vi "UHR-Fleezers Control (host) -TL FB Corrected Ronen.vi"(0 "Tab Control":T5(tab)=enum."DAQ AI") -> ()   [LabVIEW 2013] (continued)
        n1853 = Array Subset(array=w2653, index (col)=0 ("index"), length (col)=w2642) -> (w2652:dbl[][])  [unwired: 2 in]
        n1854 = Array Subset(array=w2653, index (col)=w2642) -> (w2650:dbl[][])  [unwired: 3 in]
        n1855 = Array Subset(array=w2727, index (col)=0 ("index"), length (col)=w2642) -> (w2726:dbl[][])  [unwired: 2 in]
        n1856 = Array Subset(array=w2727, index (col)=w2642) -> (w2724:dbl[][])  [unwired: 3 in]
        n1857 = Array Subset(array=w2710, index (col)=0 ("index"), length (col)=w2642) -> (w2715:dbl[][])  [unwired: 2 in]
        n1858 = Array Subset(array=w2710, index (col)=w2642) -> (w2713:dbl[][])  [unwired: 3 in]
        n1859 = for {
          tunnel: w2722 -> [w2764] mode=indexing
          tunnel: [w2763] -> w2721 mode=indexing
          workers-P: _ -> [_]
          n1860 = Reverse 1D Array(array=w2764) -> (reversed array=w2763:dbl[])
        }
        n1861 = for {
          tunnel: w2708 -> [w2760] mode=indexing
          tunnel: [w2759] -> w2707 mode=indexing
          workers-P: _ -> [_]
          n1862 = Reverse 1D Array(array=w2760) -> (reversed array=w2759:dbl[])
        }
        n1863 = for {
          tunnel: w2652 -> [w2758] mode=indexing
          tunnel: [w2757] -> w2651 mode=indexing
          workers-P: _ -> [_]
          n1864 = Reverse 1D Array(array=w2758) -> (reversed array=w2757:dbl[])
        }
        n1865 = for {
          tunnel: w2726 -> [w2766] mode=indexing
          tunnel: [w2765] -> w2725 mode=indexing
          workers-P: _ -> [_]
          n1866 = Reverse 1D Array(array=w2766) -> (reversed array=w2765:dbl[])
        }
        n1867 = for {
          tunnel: w2715 -> [w2762] mode=indexing
          tunnel: [w2761] -> w2714 mode=indexing
          workers-P: _ -> [_]
          n1868 = Reverse 1D Array(array=w2762) -> (reversed array=w2761:dbl[])
        }
        n1869 = Index Array(array=w2727, index (row)=0) -> (element=→"Waveform Graph":dbl[])  [unwired: 1 in]
        n1870 = Add(x=w2721, y=w2720) -> (x+y=w2719:dbl[][])
        n1871 = Add(x=w2707, y=w2706) -> (x+y=w2705:dbl[][])
        n1872 = Add(x=w2651, y=w2650) -> (x+y=w2635:dbl[][])
        n1873 = Add(x=w2725, y=w2724) -> (x+y=w2699:dbl[][])
        n1874 = Add(x=w2714, y=w2713) -> (x+y=w2712:dbl[][])
        n1875 = Divide(x=w2705, y=2) -> (x/y=w2703:dbl[][])
        n1876 = Divide(x=w2719, y=2) -> (x/y=w2664:dbl[][])
        n1877 = Divide(x=w2712, y=2) -> (x/y=w2666:dbl[][])
        n1878 = To Single Precision Float(number=w2699) -> (single precision float=w2698:sgl[][])
        n1879 = Transpose 2D Array(2D array=w2703) -> (transposed array=→"Data map":dbl[][])
        n1880 = To Single Precision Float(number=w2635) -> (single precision float=w2639:sgl[][])
        n1881 = To Single Precision Float(number=w2664) -> (single precision float=w2670:sgl[][])
        n1882 = To Single Precision Float(number=w2666) -> (single precision float=w2667:sgl[][])
        n1883 = call "IMAQ ArrayToImage"("Image Pixels (Float)"=w2698, "Image"=w2632) -> ("Image Out"=w2701:T3)  [unwired: 8 in, 1 out]
        n1884 = call "IMAQ ArrayToImage"("Image Pixels (Float)"=w2639, "Image"=w2631) -> ("Image Out"=w2641:T3)  [unwired: 8 in, 1 out]
        n1885 = call "IMAQ ArrayToImage"("Image Pixels (Float)"=w2670, "Image"=w2630) -> ("Image Out"=w2672:T3)  [unwired: 8 in, 1 out]
        n1886 = call "IMAQ ArrayToImage"("Image Pixels (Float)"=w2667, "Image"=w2629) -> ("Image Out"=w2669:T3)  [unwired: 8 in, 1 out]
        n1887 = call "IMAQ Symmetry"("Type of Symmetry"=w2700, "Image Src"=w2701) -> ("Image Dst Out"=w2696:T3)  [unwired: 3 in, 1 out]
        n1888 = call "IMAQ Symmetry"("Type of Symmetry"=w2640, "Image Src"=w2641) -> ("Image Dst Out"=w2637:T3)  [unwired: 3 in, 1 out]
        n1889 = call "IMAQ Symmetry"("Type of Symmetry"=w2671, "Image Src"=w2672) -> ("Image Dst Out"=→"Detection Laser X":T3)  [unwired: 3 in, 1 out]
        n1890 = call "IMAQ Symmetry"("Type of Symmetry"=w2668, "Image Src"=w2669) -> ("Image Dst Out"=→"Detection Laser Y":T3)  [unwired: 3 in, 1 out]
        n1891 = call "IMAQ Set Simple Calibration"("Calibration Axis Info"=T37 {"Origin Pixel"={"X"=0.0, "Y"=0.0}, "Angle Relative to Horizontal (deg)"=0.0, "Axis Reference"=0}, "Grid Descriptor"=T38 {"X Step"=0.3, "Y Step"=0.3, "Unit"=enum."Undefined"}, "Image"=w2696) -> ("Calibrated Image"=→"APD 1":T3)  [unwired: 7 in, 1 out]
        n1892 = call "IMAQ Set Simple Calibration"("Calibration Axis Info"=T37 {"Origin Pixel"={"X"=0.0, "Y"=0.0}, "Angle Relative to Horizontal (deg)"=0.0, "Axis Reference"=0}, "Grid Descriptor"=T38 {"X Step"=0.3, "Y Step"=0.3, "Unit"=enum."Undefined"}, "Image"=w2637) -> ("Calibrated Image"=→"APD 2":T3)  [unwired: 7 in, 1 out]
      }
    }
    n1893 = Subtract(x=w2222, y="APD 2 Offset") -> (x-y=w2219:waveform(dbl))
    n1894 = Subtract(x=w2224, y="APD 1 Offset") -> (x-y=w2220:waveform(dbl))
    n1895 = Index Array(array=w2239, index=3) -> (element=w2307:waveform(dbl))
    n1896 = Index Array(array=w2239, index=6) -> (element=w2304:waveform(dbl))
    n1897 = Build Array(w2220, w2219) -> (→"APD Chart":waveform(dbl)[])
    n1898 = Array Size(array=w2297) -> (size(s)=w2347:i32)
    n1899 = call <vilib>:"Std Deviation and Variance.vi"("X"=w2232) -> ("standard deviation"=w2231:dbl)  [unwired: 1 in, 2 out]
    n1900 = Add Array Elements(numeric array=w2232) -> (sum=w2234:u32)
    n1901 = Add Array Elements(numeric array=w2297) -> (sum=w2357:u32)
    n1902 = call <vilib>:"Std Deviation and Variance.vi"("X"=w2297) -> ("standard deviation"=w2296:dbl)  [unwired: 1 in, 2 out]
    n1903 = Divide(x=w2231, y=w2230) -> (x/y=w2227:dbl)
    "Rate sigma (Hz) 2" <- w2227
    n1904 = Multiply(x=w2230, y=w2347) -> (x*y=w2233:dbl)
    "Int. Time (s)" <- w2233
    n1905 = Divide(x=w2234, y=w2233) -> (x/y=w2228:dbl)
    "APD 2 Rate (Hz)" <- w2228
    n1906 = Divide(x=w2357, y=w2233) -> (x/y=w2294:dbl)
    "APD 1 Rate (Hz)" <- w2294
    n1907 = Divide(x=w2296, y=w2230) -> (x/y=w2295:dbl)
    "Rate sigma (Hz)" <- w2295
    n1908 = Divide(x=w2227, y=w2228) -> (x/y=→"Sigma/Mean 2":dbl)
    n1909 = Divide(x=w2295, y=w2294) -> (x/y=→"Sigma/Mean":dbl)
    n1910 = case shown="2" "Calibration" {
      tunnel: "T1 alpha_x (nm/V)" -> [_ w2595 w2616]
      tunnel: "T1 kappa_x (pN/nm)" -> [_ _ w2606]
      tunnel: "T2 alpha_x (nm/V)" -> [_ w2594 w2614]
      tunnel: "T2 kappa_x (pN/nm)" -> [_ _ w2607]
      tunnel: w2307 -> [w2577 w2592 w2612]
      tunnel: w2304 -> [w2576 w2590 w2610]
      tunnel: [w2577 w2589 w2609] -> w2333
      tunnel: [w2576 w2588 w2608] -> w2332
      tunnel: ["T1 X (V)" ("Label.Text") "T1 X (nm)" ("Label.Text") "T1 X (pN)" ("Label.Text")] -> w2325
      tunnel: ["T2 X (V)" ("Label.Text") "T2 X (nm)" ("Label.Text") "T2 X (pN)" ("Label.Text")] -> w2324
      tunnel: ["Position (V)" ("Label.Text") "Position (nm)" ("Label.Text") "Force (pN)" ("Label.Text")] -> w2326
      tunnel: w2306 -> [_ w2580 w2599]
      tunnel: w2308 -> [_ w2583 w2601]
      tunnel: ["Mean (V)" ("Label.Text") "Mean (nm)" ("Label.Text") "Mean (pN)" ("Label.Text")] -> w2321
      tunnel: ["Difference (V)" ("Label.Text") "Difference (nm)" ("Label.Text") "Difference (pN)" ("Label.Text")] -> w2247
      frame 0, Default {
      }
      frame 1 {
        # "position"
        n1911 = Unbundle By Name(w2592) -> ("Y"=w2596:dbl[])
        n1912 = Unbundle By Name(w2590) -> ("Y"=w2581:dbl[])
        n1913 = Subtract(x=w2596, y=w2583) -> (x-y=w2584:dbl[])
        n1914 = Subtract(x=w2581, y=w2580) -> (x-y=w2582:dbl[])
        n1915 = Multiply(x=w2582, y=w2594) -> (x*y=w2591:dbl[])
        n1916 = Multiply(x=w2595, y=w2584) -> (x*y=w2593:dbl[])
        n1917 = Bundle By Name(cluster=w2590, "Y"=w2591) -> (w2588:waveform(dbl))
        n1918 = Bundle By Name(cluster=w2592, "Y"=w2593) -> (w2589:waveform(dbl))
      }
      frame 2 {
        # "force"
        n1919 = Unbundle By Name(w2612) -> ("Y"=w2617:dbl[])
        n1920 = Unbundle By Name(w2610) -> ("Y"=w2615:dbl[])
        n1921 = Subtract(x=w2615, y=w2599) -> (x-y=w2600:dbl[])
        n1922 = Subtract(x=w2617, y=w2601) -> (x-y=w2602:dbl[])
        n1923 = Compound Arithmetic op=MULTIPLY(w2600, w2614, w2607) -> (w2611:dbl[])
        n1924 = Compound Arithmetic op=MULTIPLY(w2606, w2616, w2602) -> (w2613:dbl[])
        n1925 = Bundle By Name(cluster=w2610, "Y"=w2611) -> (w2608:waveform(dbl))
        n1926 = Bundle By Name(cluster=w2612, "Y"=w2613) -> (w2609:waveform(dbl))
      }
    }
    n1927 = feedback-in #17("Calibration") -> ()
    n1928 = feedback #17(u16 1 ("Calibration")) -> (w2328:u16)
    n1929 = local read "Trap 2 Bead Size (nm)"() -> (w2127:dbl)
    n1930 = local read "Trap 1 Bead Size (nm)"() -> (w2126:dbl)
    n1931 = local read "AOM X Cal (nm/MHz)"() -> (w2124:dbl)
    n1932 = local read "Trap Delta (MHz)"() -> (w2123:dbl)
    n1933 = Not Equal?(x=w2328, y="Calibration") -> (x != y?=w2285:bool)
    n1934 = Multiply(x=w2124, y=w2123) -> (x*y=w2128:dbl)
    n1935 = Add(x=w2127, y=w2126) -> (x+y=w2130:dbl)
    n1936 = Unbundle By Name(w2307) -> ("Y"=w2310:dbl[])
    n1937 = Unbundle By Name(w2304) -> ("Y"=w2313:dbl[])
    n1938 = Divide(x=w2130, y=2.0) -> (x/y=w2125:dbl)
    n1939 = Subtract(x=w2310, y=w2308) -> (x-y=w2311:dbl[])
    n1940 = Subtract(x=w2313, y=w2306) -> (x-y=w2312:dbl[])
    n1941 = disable-structure shown="Enabled" {
      disable-tunnel: [-1.0 ("y") 1.0] -> w2314
      frame Disabled {
      }
      frame Enabled {
      }
    }
    n1942 = Multiply(x=w2312, y="T2 alpha_x (nm/V)") -> (x*y=w2303:dbl[])
    n1943 = Multiply(x="T1 alpha_x (nm/V)", y=w2311) -> (x*y=w2302:dbl[])
    n1944 = Multiply(x=w2332, y=w2314) -> (x*y=w2315:waveform(dbl))
    n1945 = case shown="False" "Read Lateness and Rel Phase" {
      tunnel: w2106 -> [w2543 w2565]
      tunnel: w2139 -> [w2544 w2564]
      tunnel: [w2543 w2563] -> w2300
      tunnel: [w2544 w2562] -> w2299
      frame False {
      }
      frame True {
        n1946 = xnode "Read/Write Control"("FPGA VI Reference In"=w2565, "error in"=w2564) -> ("FPGA VI Reference Out"=w2563:T20, "error out"=w2562:errorcluster, "GI Relative phase"=→"GI relative phase":i16, "Relative phase"=→"Relative phase (AI1)":i16, "AI Late Counter"=→"Late Counter (AI1)":u16, "GI Late Counter"=→"GI Late Counter":u16, "MCL Late Counter"=→"MCL Late Counter":u16, "MCL Relative Phase"=→"Relative Phase (MCL)":i16, "APD Acq Relative Phase"=→"APD Acq Relative Phase":i16, "APD 1 Gate Relative Phase"=→"APD 1 Gate Relative Phase":i16, "APD 2 Gate Relative Phase"=→"APD 2 Gate Relative Phase":i16, "APD Acq Late Counter"=→"APD Acq Late Counter":u16, "APD 1 Gate Late Counter"=→"APD 1 Gate Late Counter":u16, "APD 2 Gate Late Counter"=→"APD 2 Gate Late Counter":u16, "Green FB Relative Phase"=→"Relative phase (Green FB)":i16, "GI Relative phase 2"=→"GI relative phase 2":i16, "GI Late Counter 2"=→"GI Late Counter 2":u16, "Trap Pos FIFO Timeout"=→"Trap Pos FIFO Timeout":u16, "Trap AI FIFO Timeout"=→"Trap AI FIFO Timeout":u16)
      }
    }
    n1947 = Subtract(x=w2303, y=w2302) -> (x-y=w2122:dbl[])
    n1948 = call-poly <vilib>:"Mean.vi"("X"=w2122) -> ("mean"=w2129:dbl)  [unwired: 1 out]
    n1949 = Add(x=w2128, y=w2129) -> (x+y=w2132:dbl)
    n1950 = Subtract(x=w2132, y=w2125) -> (x-y=→"Tether Extension (nm, calculated)":dbl)
    n1951 = Unbundle By Name(w2332) -> ("Y"=w2272:dbl[])
    n1952 = Unbundle By Name(w2333) -> ("Y"=w2273:dbl[])
    n1953 = Build Array(w2333, w2315) -> (→"Force":waveform(dbl)[])
    n1954 = Subtract(x=w2122, y="Offset (nm)") -> (x-y=w2270:dbl[])
    n1955 = call-poly <vilib>:"Mean.vi"("X"=w2272) -> ("mean"=w2251:dbl)  [unwired: 1 out]
    "T2 X" <- w2251
    n1956 = Absolute Value(x=w2273) -> (abs(x)=w2274:dbl[])
    n1957 = Absolute Value(x=w2272) -> (abs(x)=w2275:dbl[])
    n1958 = call-poly <vilib>:"Mean.vi"("X"=w2273) -> ("mean"=w2252:dbl)  [unwired: 1 out]
    "T1 X" <- w2252
    n1959 = Add(x=w2274, y=w2275) -> (x+y=w2276:dbl[])
    n1960 = Bundle By Name(cluster=w2307, "Y"=w2270) -> (w2238:waveform(dbl))
    "Bead Separation" <- w2238
    n1961 = Divide(x=w2276, y=2.0) -> (x/y=→"Vec Mean of T1 T2":dbl[])
    n1962 = case shown="True" w2285 {
      tunnel: w2326 -> [_ w2570]
      tunnel: w2325 -> [_ w2569]
      tunnel: w2324 -> [_ w2568]
      tunnel: w2321 -> [_ w2567]
      tunnel: w2247 -> [_ w2566]
      frame False {
      }
      frame True {
        n1963 = property on="Force" class="WFChart (strict)"("YScale.NameLbl.Text"=w2570) -> ()  [unwired: 2 in, 2 out]
        n1964 = property on="T2 X" class="DigNum (strict)"("Caption.Text"=w2568) -> ()  [unwired: 2 in, 2 out]
        n1965 = property on="T1 X" class="DigNum (strict)"("Caption.Text"=w2569) -> ()  [unwired: 2 in, 2 out]
        n1966 = property on="Mean" class="DigNum (strict)"("Caption.Text"=w2567) -> ()  [unwired: 2 in, 2 out]
        n1967 = property on="Difference" class="DigNum (strict)"("Caption.Text"=w2566) -> ()  [unwired: 2 in, 2 out]
      }
    }
    n1968 = local read "Tether"() -> (w2279:bool)
    n1969 = Absolute Value(x=w2252) -> (abs(x)=w2249:dbl)
    n1970 = Absolute Value(x=w2251) -> (abs(x)=w2248:dbl)
    n1971 = Add(x=w2249, y=w2248) -> (x+y=w2323:dbl)
    n1972 = Subtract(x=w2249, y=w2248) -> (x-y=→"Difference":dbl)
    n1973 = feedback #18(w2270) -> (w2269:dbl[])
    n1974 = Divide(x=w2323, y=2.0) -> (x/y=w2278:dbl)
    "Mean" <- w2278
    n1975 = case shown="True" w2279 {
      tunnel: w2278 -> [_ w2502]
      frame False {
      }
      frame True {
        n1976 = Greater?(x="Lost Tether Alarm Threshold (pN)", y=w2502) -> (0:w2500:bool)
        n1977 = case shown="True" w2500 {
          frame False {
          }
          frame True {
            n1978 = flat-sequence {
              frame #0 {
                # "stop only if saving"
                n1979 = local read "Saving..."() -> (w2515:bool)
                n1980 = And(x=w2515, y="TA Cancel Save?") -> (x .and. y?=w2514:bool)
                n1981 = local write "Stop Saving"(w2514) -> ()
              }
              frame #1 {
                n1982 = case shown="True" "TA Green Off?" {
                  frame False {
                  }
                  frame True {
                    w2518 = FALSE ("Fl. Triggered...")
                    n1983 = local write "Fl. Triggered..."(w2518) -> ()
                    n1984 = property on="Green Laser ON/Interlacing" class="Bool (strict)"("Val(Sgnl)"=w2518) -> ()  [unwired: 2 in, 2 out]
                  }
                }
              }
            }
            n1985 = local read "Time tether formed"() -> (w2509:timestamp)
            n1986 = Get Date/Time In Seconds() -> (seconds since 1Jan1904=w2510:timestamp)
            n1987 = Subtract(x=w2510, y=w2509) -> (x-y=w2508:dbl)
            n1988 = Number To Decimal String(number=w2508) -> (decimal integer string=w2505:string)  [unwired: 1 out]
            n1989 = local read "Messages"() -> (w2512:string)
            n1990 = call <vilib>:"Beep.vi"() -> ()  [unwired: 3 in, 9 out]
            n1991 = Concatenate Strings("Lost tether (" ("Message to add"), w2505, " s)." ("string")) -> (w2507:string)
            n1992 = local write "Tether"(FALSE ("Tether")) -> ()
            n1993 = call "Update messages.vi"("Message to add"=w2507, "Old message string"=w2512) -> ("New message string"=w2511:string)
            n1994 = local write "Messages"(w2511) -> ()
            n1995 = property on="Trap Pos. FB ON" class="Bool (strict)"("Val(Sgnl)"=FALSE ("Value (Signaling)")) -> ()  [unwired: 2 in, 2 out]
          }
        }
      }
    }
    n1996 = Build Array (concatenate)(w2270, w2269) -> (w2268:dbl[])
    n1997 = Split 1D Array(array=w2268, index=w2150) -> (first subarray=w2264:dbl[])  [unwired: 1 out]
    n1998 = feedback-in #18(w2264) -> ()
    n1999 = call-poly <vilib>:"Mean.vi"("X"=w2264) -> ("mean"=w2263:dbl)  [unwired: 1 out]
    "Bead Mean (nm)" <- w2263
    n2000 = Subtract(x=w2264, y=w2263) -> (x-y=w2262:dbl[])
    n2001 = Square(x=w2262) -> (x^2=w2261:dbl[])
    n2002 = call-poly <vilib>:"Mean.vi"("X"=w2261) -> ("mean"=w2260:dbl)  [unwired: 1 out]
    n2003 = Square Root(x=w2260) -> (sqrt(x)=w2259:dbl)
    n2004 = Multiply(x=10.0, y=w2259) -> (x*y=→"RMS (Ang)":dbl)
    n2005 = xnode "Read/Write Control"("FPGA VI Reference In"=w2300, "error in"=w2299) -> ("FPGA VI Reference Out"=w2411:T20, "error out"=w2405:errorcluster, "AI4 Y Sum Set 1"=w2401:i16, "AI4 Y Sum Set 2"=w2400:i16, "AI1 X Set 1"=w2184:fxp<+/-,16,1>, "AI1 X Set 2"=w2183:fxp<+/-,16,1>, "Trap Pos FB Int Signal"=→"Trap Pos FB Int Signal":fxp<+/-,24,9>, "Trap Pos FB Int-Norm Signal"=→"Trap Pos FB Int-Norm Signal":fxp<+/-,24,9>, "Trap Pos FB Action"=w2177:i64, "Scanning"=→"AOD Scanning":bool, "Scan I"=→"AOD Scan I":u64, "Scanning MCL"=w2403:bool, "Scan I (MCL)"=→"MCL Scan I":u64, "Green FB Signals"=w2342:T48)  [unwired: 1 out]
    "MCL Scanning" <- w2403
    "Trap Pos FB Action" <- w2177
    n2006 = local read "AI2 (V)"() -> (w2402:cluster{"Set 1":dbl, "Set 2":dbl})
    n2007 = Bundle By Name(cluster=w2402, "Set 1"=w2401, "Set 2"=w2400) -> (w2398:cluster{"Set 1":dbl, "Set 2":dbl})
    n2008 = Divide(x=w2177, y=327.67) -> (x/y=→"Action (%)":dbl)
    n2009 = local read "Trap X (AI1)"() -> (w2197:T1)
    n2010 = Divide(x=w2398, y=3276.7) -> (x/y=w2397:cluster{"Set 1":dbl, "Set 2":dbl})
    n2011 = local write "AI2 (V)"(w2397) -> ()
    n2012 = Bundle(cluster=w2197, "Trap 1"=w2184, "Trap 2"=w2183) -> (→"Trap X (AI1)":T1)
    n2013 = Divide(x=w2342, y=3276.7) -> (x/y=w2338:T49)
    n2014 = Unbundle By Name(w2338) -> ("Green FB Ch 0"=w2341:dbl, "Green FB Ch 1"=w2340:dbl, "Green FB Ch 2"=w2339:dbl)
    n2015 = Divide(x=w2341, y=w2339) -> (x/y=w2337:dbl)
    n2016 = Divide(x=w2340, y=w2339) -> (x/y=w2336:dbl)
    n2017 = flat-sequence "To save data" {
      tunnel: [w3392] -> w2422
      tunnel: [w3393] -> w2421
      tunnel: w2373 -> [w3386]
      tunnel: w2266 -> [w3390]
      tunnel: ["Save Calibration"] -> w2394
      tunnel: w2391 -> [w3389]
      tunnel: [w3382] -> w2390
      tunnel: [w3379] -> w2389
      tunnel: [w3376] -> w2388
      tunnel: w2372 -> [w3378]
      tunnel: w2283 -> [w3372]
      tunnel: [w3372] -> w2282
      tunnel: ["Start Saving"] -> w2240
      tunnel: [w3366] -> w2166
      tunnel: [w3365] -> w2165
      tunnel: w2422 -> [w3627]
      tunnel: w2421 -> [w3626]
      tunnel: w2167 -> [w3625]
      tunnel: w2394 -> [w3624]
      tunnel: w2390 -> [w3622]
      tunnel: w2389 -> [w3621]
      tunnel: w2388 -> [w3620]
      tunnel: w2253 -> [w3619]
      tunnel: w2292 -> [w3618]
      tunnel: w2282 -> [w3617]
      tunnel: w2240 -> [w3616]
      tunnel: w2238 -> [w3615]
      tunnel: w2214 -> [w3614]
      tunnel: w2166 -> [w3613]
      tunnel: w2165 -> [w3612]
      tunnel: w2164 -> [w3611]
      frame #0 {
        n2018 = Or(x="Save N Sets", y="Start Saving") -> (x .or. y?=w3373:bool)
        n2019 = To Double Precision Float(number=w3389) -> (double precision float=w3383:dbl)
        n2020 = Build Array(w3373, "Save Calibration", w3386, w3378) -> (w3388:bool[])
        n2021 = Compound Arithmetic op=OR("Save Calibration", w3386, w3373, w3378) -> (w3391:bool)
        n2022 = Boolean Array To Number(Boolean array=w3388) -> (number=w3385:u32)
        n2023 = feedback #19(FALSE ("Save APD Data\nwith Trap Data")) -> (w3367:bool)
        n2024 = feedback #20(refnum<k0> refnum) -> (w3394:refnum<file>)
        n2025 = feedback #21(refnum<k0> refnum) -> (w3369:refnum<file>)
        n2026 = feedback #22(FALSE ("Save APD Data\nwith Trap Data")) -> (w3377:bool)
        n2027 = feedback #23(refnum<k0> refnum) -> (w3380:refnum<file>)
        n2028 = feedback #24(0) -> (w3396:i32)
        n2029 = feedback #25() -> (w3384:u32)  [unwired: 1 out]
        n2030 = case shown="True" w3391 {
          tunnel: [w3403 1] -> w3392
          tunnel: w3396 -> [w3405 _]
          tunnel: [w3404 w3423] -> w3393
          tunnel: w3394 -> [w3404 _]
          tunnel: w3390 -> [_ w3443]
          tunnel: w3383 -> [_ w3441]
          tunnel: w3385 -> [_ w3444]
          tunnel: [w3402 w3422] -> w3382
          tunnel: w3384 -> [w3402 _]
          tunnel: [w3401 w3420] -> w3379
          tunnel: w3380 -> [w3401 _]
          tunnel: [w3400 w3419] -> w3376
          tunnel: w3377 -> [w3400 _]
          tunnel: "Start Saving" -> [_ w3417]
          tunnel: w3372 -> [_ w3416]
          tunnel: [w3399 w3407] -> w3365
          tunnel: w3369 -> [w3399 _]
          tunnel: [w3398 w3406] -> w3366
          tunnel: w3367 -> [w3398 _]
          frame False {
            n2031 = Increment(x=w3405) -> (x+1=w3403:i32)
          }
          frame True {
            w3413 = FALSE ("Start Saving")
            w3418 = 9.0  # File Version
            w3426 = FALSE ("prepend array or string size? (T)")
            w3424 = T30."big-endian, network order" ("byte order (0:big-endian, network order)")
            # "write file headers"
            n2032 = local read "BD 1 Frequency 1 (MHz)"() -> (w3440:dbl)
            n2033 = local read "BD 2 Frequency 1 (MHz)"() -> (w3439:dbl)
            n2034 = local read "BD 1 Frequency 2 (MHz)"() -> (w3438:dbl)
            n2035 = local read "BD 2 Frequency 2 (MHz)"() -> (w3437:dbl)
            n2036 = local read "BD 1 Frequency 3 (MHz)"() -> (w3436:dbl)
            n2037 = local read "BD 2 Frequency 3 (MHz)"() -> (w3435:dbl)
            n2038 = Array Size(array=w3416) -> (size(s)=w3415:i32)
            n2039 = To Double Precision Float(number=w3415) -> (double precision float=w3414:dbl)
            n2040 = local write "Save Calibration"(w3413) -> ()
            n2041 = local write "Start Saving"(w3413) -> ()
            n2042 = Build Array("Save APD Data\nwith Trap Data", "Save Trap Pos. Data") -> (w3410:bool[])
            n2043 = Boolean Array To Number(Boolean array=w3410) -> (number=w3409:u32)
            n2044 = Build Array(w3440, w3439, w3438, w3437, w3436, w3435) -> (w3434:dbl[])
            n2045 = case shown="4" w3444 {
              tunnel: w3443 -> [w3515 w3535 w3551 w3589]
              tunnel: w3414 -> [w3520 w3542 w3571 w3608]
              tunnel: w3441 -> [w3519 w3541 w3570 w3607]
              tunnel: [w3516 w3537 w3562 w3599] -> w3432
              tunnel: [w3507 "Cal sets to save" w3552 w3590] -> w3422
              tunnel: w3434 -> [w3517 w3538 w3564 w3601]
              tunnel: "Save APD Data\nwith Trap Data" -> [w3514 _ w3548 w3587]
              tunnel: [w3514 w3529 w3548 w3587] -> w3419
              tunnel: w3418 -> [w3510 w3530 w3546 w3585]
              tunnel: w3417 -> [w3509 _ _ _]
              tunnel: [w3500 w3529 w3545 w3575] -> w3406
              tunnel: "Save Trap Pos. Data" -> [w3500 _ w3545 w3575]
              tunnel: w3409 -> [w3499 _ w3544 w3574]
              frame 1, Default {
                # "timeseries"
                n2046 = case shown="True" "Profile" {
                  tunnel: [w3523 w3526] -> w3504
                  tunnel: [w3523 w3525] -> w3503
                  tunnel: [w3523 w3524] -> w3502
                  tunnel: [w3523 w3528] -> w3501
                  frame False {
                    w3523 = 0.0 ("f")
                  }
                  frame True {
                    n2047 = local read "Current Position"() -> (w3527:dbl[])
                    n2048 = local read "Y change (mm)"() -> (w3528:dbl)
                    n2049 = call "subVI_explode3array.vi"("Array"=w3527) -> ("x"=w3526:dbl, "y"=w3525:dbl, "z"=w3524:dbl)  [unwired: 12 in]
                  }
                }
                n2050 = local read "Save ave N"() -> (w3522:dbl)
                n2051 = Multiply(x=w3522, y=w3515) -> (x*y=w3521:dbl)
                n2052 = To Double Precision Float(number=w3499) -> (double precision float=w3513:dbl)
                n2053 = Build Array(w3510, w3515, w3521, w3520, w3519, 0.0 ("f")) -> (w3518:dbl[])
                n2054 = Build Array(w3513, w3504, w3503, w3502, w3501) -> (w3511:dbl[])
                n2055 = Select(t=u32 4000000000, s=w3509, f="N sets to save") -> (s? t:f=w3507:u32)
                n2056 = Build Array (concatenate)(w3518, w3517, w3511) -> (w3516:dbl[])
              }
              frame 2 {
                w3532 = 0.0 ("f")
                w3529 = FALSE ("Save APD Data\nwith Trap Data")
                # "calibration"
                n2057 = Boolean To (0,1)(Boolean=w3529) -> (0, 1=w3534:i16)
                n2058 = To Double Precision Float(number=w3534) -> (double precision float=w3533:dbl)
                n2059 = Build Array(w3533, w3532, w3532, w3532, w3532) -> (w3531:dbl[])
                n2060 = Build Array(w3530, w3535, w3535, w3542, w3541, 1.0 ("t")) -> (w3539:dbl[])
                n2061 = Build Array (concatenate)(w3539, w3538, w3531) -> (w3537:dbl[])
                "Calibrating Trap..." <- TRUE ("Calibrating...")
              }
              frame 4 {
                w3549 = 0.0 ("f")
                # "write file header for a trap \nraster scan"
                # "scan dir (x/y = 0/1)"
                # "cycles/step"
                # "n scans (f/b)"
                # "steps"
                # "freq. range"
                # "AOD raster scan"
                n2062 = local read "Number of F/B Scans (AOD)"() -> (w3556:u16)
                n2063 = local read "Cycles/step (AOD)"() -> (w3558:u64)
                n2064 = local read "Scan Range (MHz)"() -> (w3561:dbl)
                n2065 = local read "Scan steps (AOD)"() -> (w3560:u64)
                n2066 = local read "Scan BD"() -> (w3568:bool)
                n2067 = local read "Save ave N"() -> (w3573:dbl)
                n2068 = Boolean To (0,1)(Boolean=w3568) -> (0, 1=w3567:i16)
                n2069 = To Double Precision Float(number=w3556) -> (double precision float=w3555:dbl)
                n2070 = To Double Precision Float(number=w3560) -> (double precision float=w3559:dbl)
                n2071 = To Double Precision Float(number=w3558) -> (double precision float=w3557:dbl)
                n2072 = To Double Precision Float(number=w3567) -> (double precision float=w3566:dbl)
                n2073 = Multiply(x=w3573, y=w3551) -> (x*y=w3572:dbl)
                n2074 = To Double Precision Float(number=w3544) -> (double precision float=w3550:dbl)
                n2075 = Build Array(w3550, w3549, w3549, w3549, w3549) -> (w3547:dbl[])
                n2076 = local read "N sets should be saved"() -> (w3553:dbl)
                n2077 = Build Array(w3566, w3561, w3559, w3557, w3555) -> (w3563:dbl[])
                n2078 = Build Array(w3546, w3551, w3572, w3571, w3570, 2.0 ("t")) -> (w3565:dbl[])
                n2079 = Round Toward +Infinity(x=w3553) -> (ceil(x): smallest int >= x=w3554:dbl)
                n2080 = Build Array (concatenate)(w3565, w3564, w3547, w3563) -> (w3562:dbl[])
                n2081 = To Unsigned Long Integer(number=w3554) -> (unsigned 32bit integer=w3552:u32)
              }
              frame 8 {
                w3582 = 0.0 ("f")
                # "MCL raster scan"
                n2082 = local read "Number of scans (MCL)"() -> (w3577:u64)
                n2083 = local read "Scan lines (y)"() -> (w3576:u64)
                n2084 = local read "2D or 1D Scan"() -> (w3579:bool)
                n2085 = local read "Scan Range (V)\n(of steps)"() -> (w3598:dbl)
                n2086 = local read "Fast Scan Dir"() -> (w3605:bool)
                n2087 = local read "Cycles/step (MCL)"() -> (w3595:u64)
                n2088 = local read "Scan steps (MCL)"() -> (w3597:u64)
                n2089 = Select(t=w3576, s=w3579, f=w3577) -> (s? t:f=w3578:u64)
                n2090 = Boolean To (0,1)(Boolean=w3579) -> (0, 1=w3581:i16)
                n2091 = local read "Save ave N"() -> (w3610:dbl)
                n2092 = local read "Initial X"() -> (w3584:dbl)
                n2093 = local read "Initial Y"() -> (w3583:dbl)
                n2094 = To Double Precision Float(number=w3581) -> (double precision float=w3580:dbl)
                n2095 = Boolean To (0,1)(Boolean=w3605) -> (0, 1=w3604:i16)
                n2096 = To Double Precision Float(number=w3578) -> (double precision float=w3593:dbl)
                n2097 = To Double Precision Float(number=w3597) -> (double precision float=w3596:dbl)
                n2098 = To Double Precision Float(number=w3595) -> (double precision float=w3594:dbl)
                n2099 = To Double Precision Float(number=w3604) -> (double precision float=w3603:dbl)
                n2100 = Multiply(x=w3610, y=w3589) -> (x*y=w3609:dbl)
                n2101 = To Double Precision Float(number=w3574) -> (double precision float=w3588:dbl)
                n2102 = local read "N sets should be saved (MCL)"() -> (w3591:dbl)
                n2103 = Build Array(w3588, w3580, w3582, w3582, w3582) -> (w3586:dbl[])
                n2104 = Build Array(w3603, w3598, w3596, w3594, w3593, w3584, w3583) -> (w3600:dbl[])
                n2105 = Build Array(w3585, w3589, w3609, w3608, w3607, 3.0 ("t")) -> (w3602:dbl[])
                n2106 = Round Toward +Infinity(x=w3591) -> (ceil(x): smallest int >= x=w3592:dbl)
                n2107 = Build Array (concatenate)(w3602, w3601, w3586, w3600) -> (w3599:dbl[])
                n2108 = To Unsigned Long Integer(number=w3592) -> (unsigned 32bit integer=w3590:u32)
              }
            }
            n2109 = local read "Index"() -> (w3449:dbl)
            n2110 = call "Create new save file.vi"("Insert"="", "Ext"=".dat", "Index In"=w3449) -> ("Path Out"=w3408:path, "Index Out"=w3421:dbl)
            n2111 = local write "Save file name"(w3408) -> ()
            n2112 = local write "Index"(w3421) -> ()
            n2113 = local write "Save index"(w3421) -> ()
            n2114 = Array Size(array=w3432) -> (size(s)=w3433:i32)
            n2115 = Open/Create/Replace File(file path (use dialog)=w3408, operation (0:open)=T24."create", access (0:read/write)=enum16{"read/write", "read-only", "write-only"}."write-only") -> (refnum out=w3446:refnum<file>)  [unwired: 1 in, 4 out]
            n2116 = local write "Saving..."(TRUE ("Saving...")) -> ()
            n2117 = To Double Precision Float(number=w3433) -> (double precision float=w3431:dbl)
            n2118 = String Length(string="Comment (data description)") -> (length=w3429:i32)
            n2119 = To Double Precision Float(number=w3429) -> (double precision float=w3428:dbl)
            n2120 = Deny Access(7:w3446) -> (3:w3445:refnum<file>)  [unwired: 1 in, 2 out]
            n2121 = Build Array (concatenate)(w3431, w3432, w3428) -> (w3430:dbl[])
            n2122 = case "If fluorescence data to be saved" shown="True" w3419 {
              tunnel: w3408 -> [_ w3498]
              tunnel: [refnum<k0> refnum w3478] -> w3420
              frame False {
              }
              frame True {
                w3477 = 0.0
                n2123 = local read "APD Integration Time (s)"() -> (w3483:dbl)
                n2124 = local read "N APD Samp/step"() -> (w3476:dbl)
                n2125 = Path To String(path=w3498) -> (string=w3497:string)
                n2126 = String Length(string=w3497) -> (length=w3496:i32)
                n2127 = Subtract(x=w3496, y=4) -> (x-y=w3494:i32)
                n2128 = String Subset(string=w3497, length (rest)=w3494) -> (substring=w3493:string)  [unwired: 1 out]
                n2129 = Build Array(w3483, w3476, w3477, w3477, w3477, w3477, w3477, w3477) -> (w3480:dbl[])
                n2130 = Concatenate Strings(w3493, "_fl.dat" ("string")) -> (w3491:string)
                n2131 = Array Size(array=w3480) -> (size(s)=w3482:i32)
                n2132 = String To Path(string=w3491) -> (path=w3487:path)
                n2133 = Open/Create/Replace File(file path (use dialog)=w3487, operation (0:open)=T24."create", access (0:read/write)=enum16{"read/write", "read-only", "write-only"}."write-only") -> (refnum out=w3488:refnum<file>)  [unwired: 1 in, 4 out]
                n2134 = Deny Access(7:w3488) -> (3:w3484:refnum<file>)  [unwired: 1 in, 2 out]
                n2135 = To Double Precision Float(number=w3482) -> (double precision float=w3481:dbl)
                n2136 = Build Array (concatenate)(w3481, w3480) -> (w3479:dbl[])
                n2137 = Write to Binary File(file (use dialog)=w3484, data=w3479, 5:FALSE ("prepend array or string size? (T)"), 9:T30."big-endian, network order" ("byte order (0:big-endian, network order)")) -> (refnum out=w3478:refnum<file>)  [unwired: 1 in, 3 out]
              }
            }
            n2138 = case shown="True" w3406 {
              tunnel: w3408 -> [_ w3460]
              tunnel: [refnum<k0> refnum w3459] -> w3407
              frame False {
              }
              frame True {
                w3455 = 0.0 ("element")
                n2139 = Path To String(path=w3460) -> (string=w3474:string)
                n2140 = Build Array(w3455, w3455, w3455, w3455, w3455, w3455, w3455, w3455) -> (w3456:dbl[])
                n2141 = String Length(string=w3474) -> (length=w3473:i32)
                n2142 = Subtract(x=w3473, y=4) -> (x-y=w3471:i32)
                n2143 = Array Size(array=w3456) -> (size(s)=w3458:i32)
                n2144 = String Subset(string=w3474, length (rest)=w3471) -> (substring=w3470:string)  [unwired: 1 out]
                n2145 = To Double Precision Float(number=w3458) -> (double precision float=w3457:dbl)
                n2146 = Concatenate Strings(w3470, "_pos.dat" ("string")) -> (w3468:string)
                n2147 = Build Array (concatenate)(w3457, w3456) -> (w3454:dbl[])
                n2148 = String To Path(string=w3468) -> (path=w3464:path)
                n2149 = Open/Create/Replace File(file path (use dialog)=w3464, operation (0:open)=T24."create", access (0:read/write)=enum16{"read/write", "read-only", "write-only"}."write-only") -> (refnum out=w3465:refnum<file>)  [unwired: 1 in, 4 out]
                n2150 = Deny Access(7:w3465) -> (3:w3461:refnum<file>)  [unwired: 1 in, 2 out]
                n2151 = Write to Binary File(file (use dialog)=w3461, data=w3454, 5:FALSE ("prepend array or string size? (T)"), 9:T30."big-endian, network order" ("byte order (0:big-endian, network order)")) -> (refnum out=w3459:refnum<file>)  [unwired: 1 in, 3 out]
              }
            }
            n2152 = Write to Binary File(file (use dialog)=w3445, data=w3430, 5:w3426, 9:w3424) -> (refnum out=w3427:refnum<file>)  [unwired: 1 in, 3 out]
            n2153 = Write to Binary File(file (use dialog)=w3427, data="Comment (data description)", 5:w3426, 9:w3424) -> (refnum out=w3423:refnum<file>)  [unwired: 1 in, 3 out]
          }
        }
        n2154 = feedback-in #19(w3366) -> ()
        n2155 = feedback-in #20(w3393) -> ()
        n2156 = feedback-in #21(w3365) -> ()
        n2157 = feedback-in #22(w3376) -> ()
        n2158 = feedback-in #23(w3379) -> ()
        n2159 = feedback-in #24(w3392) -> ()
        n2160 = feedback-in #25(w3382) -> ()
      }
      frame #1 {
        n2161 = local read "Saving..."() -> (w3623:bool)
        n2162 = case shown="True" w3623 {
          tunnel: w3627 -> [_ w3637]
          tunnel: w3626 -> [_ w3651]
          tunnel: w3625 -> [_ w3647]
          tunnel: w3624 -> [_ w3646]
          tunnel: w3622 -> [_ w3645]
          tunnel: w3621 -> [_ w3640]
          tunnel: w3620 -> [_ w3639]
          tunnel: w3619 -> [_ w3638]
          tunnel: w3618 -> [_ w3636]
          tunnel: w3617 -> [_ w3634]
          tunnel: w3616 -> [_ w3633]
          tunnel: w3615 -> [_ w3632]
          tunnel: w3614 -> [_ w3631]
          tunnel: w3613 -> [_ w3630]
          tunnel: w3612 -> [_ w3629]
          tunnel: w3611 -> [_ w3628]
          frame False {
          }
          frame True {
            n2163 = Multiply(x=w3637, y=w3636) -> (x*y=→"Time (s)":dbl)
            n2164 = Less Or Equal?(x=w3637, y=w3645) -> (x <= y?=w3649:bool)
            n2165 = Or(x="Stop Saving", y="Abort save 2") -> (x .or. y?=w3641:bool)
            n2166 = Not(x=w3641) -> (.not. x?=w3650:bool)
            n2167 = And(x=w3649, y=w3650) -> (x .and. y?=w3648:bool)
            n2168 = case shown="True" w3648 {
              tunnel: w3651 -> [w3658 w3726]
              tunnel: [0.0 w3729] -> w3644
              tunnel: w3637 -> [_ w3727]
              tunnel: w3645 -> [_ w3728]
              tunnel: w3647 -> [_ w3723]
              tunnel: w3646 -> [_ _]
              tunnel: w3640 -> [w3656 w3716]
              tunnel: w3639 -> [w3655 w3717]
              tunnel: w3638 -> [_ w3715]
              tunnel: w3634 -> [_ w3714]
              tunnel: w3633 -> [_ w3668]
              tunnel: w3632 -> [_ w3707]
              tunnel: w3631 -> [_ w3685]
              tunnel: w3630 -> [w3653 w3666]
              tunnel: w3629 -> [w3654 w3665]
              tunnel: w3628 -> [_ w3662]
              frame False {
                w3652 = FALSE
                n2169 = Close File(refnum=w3658) -> ()  [unwired: 1 in, 2 out]
                n2170 = case shown="True" w3655 {
                  tunnel: w3656 -> [_ w3660]
                  frame False {
                  }
                  frame True {
                    n2171 = Close File(refnum=w3660) -> ()  [unwired: 1 in, 2 out]
                  }
                }
                n2172 = case shown="True" w3653 {
                  tunnel: w3654 -> [_ w3659]
                  frame False {
                  }
                  frame True {
                    n2173 = Close File(refnum=w3659) -> ()  [unwired: 1 in, 2 out]
                  }
                }
                n2174 = local write "Calibrating Trap..."(w3652) -> ()
                n2175 = call <vilib>:"Beep.vi"() -> ()  [unwired: 3 in, 9 out]
                n2176 = local write "Stop Saving"(w3652) -> ()
                n2177 = property on="Raster Scanning..." class="Bool (strict)"("Val(Sgnl)"=w3652) -> ()  [unwired: 2 in, 2 out]
                "Saving..." <- w3652
              }
              frame True {
                n2178 = local read "Calibrating Trap..."() -> (w3718:bool)
                n2179 = case "Write fl. data" shown="True" w3717 {
                  tunnel: w3716 -> [_ w3752]
                  tunnel: w3715 -> [_ w3751]
                  frame False {
                  }
                  frame True {
                    n2180 = Write to Binary File(file (use dialog)=w3752, data=w3751, 5:FALSE ("prepend array or string size? (T)"), 9:T30."big-endian, network order" ("byte order (0:big-endian, network order)")) -> ()  [unwired: 1 in, 4 out]
                  }
                }
                n2181 = Greater?(x="Save ave N", y=1.0) -> (0:w3721:bool)
                n2182 = Not(x=w3718) -> (.not. x?=w3720:bool)
                n2183 = And(x=w3720, y=w3721) -> (x .and. y?=w3663:bool)
                n2184 = case shown="True" w3663 {
                  tunnel: w3662 -> [w3732 w3743]
                  tunnel: [w3732 w3735] -> w3661
                  tunnel: "Save ave N" -> [_ w3736]
                  frame False {
                  }
                  frame True {
                    w3733 = 2 ("dimension size")
                    n2185 = Array Size(array=w3743) -> (size(s)=w3737:i32)
                    n2186 = Divide(x=w3737, y=w3733) -> (x/y=w3741:dbl)
                    n2187 = Reshape Array(w3743, w3741, w3733) -> (w3742:u64[][])
                    n2188 = Transpose 2D Array(2D array=w3742) -> (transposed array=w3740:u64[][])
                    n2189 = for {
                      tunnel: w3740 -> [w3745] mode=indexing
                      tunnel: [w3744] -> w3734 mode=indexing
                      tunnel: w3736 -> [w3746]
                      workers-P: _ -> [_]
                      n2190 = call "downsample 1D array - U64.vi"("Ave N"=w3746, "Array In"=w3745) -> ("Array Out"=w3744:u64[])  [unwired: 1 in]
                    }
                    n2191 = Transpose 2D Array(2D array=w3734) -> (transposed array=w3739:u64[][])
                    n2192 = Divide(x=w3737, y=w3736) -> (x/y=w3738:dbl)
                    n2193 = Reshape Array(w3739, w3738) -> (w3735:u64[])
                  }
                }
                n2194 = case shown="True" w3663 {
                  tunnel: w3723 -> [w3755 w3767]
                  tunnel: [w3755 w3759] -> w3719
                  tunnel: "Save ave N" -> [_ w3760]
                  tunnel: w3714 -> [_ w3758]
                  frame False {
                    # "don't downsample data for trap calibration"
                  }
                  frame True {
                    n2195 = Array Size(array=w3767) -> (size(s)=w3761:i32)
                    n2196 = Array Size(array=w3758) -> (size(s)=w3757:i32)
                    n2197 = Divide(x=w3761, y=w3757) -> (x/y=w3765:dbl)
                    n2198 = Reshape Array(w3767, w3765, w3757) -> (w3766:i16[][])
                    n2199 = Transpose 2D Array(2D array=w3766) -> (transposed array=w3764:i16[][])
                    n2200 = for {
                      tunnel: w3764 -> [w3770] mode=indexing
                      tunnel: [w3769] -> w3756 mode=indexing
                      tunnel: w3760 -> [w3768]
                      workers-P: _ -> [_]
                      n2201 = call "downsample 1D array - I16.vi"("Ave N"=w3768, "Array In"=w3770) -> ("Array Out"=w3769:i16[])  [unwired: 1 out]
                    }
                    n2202 = Transpose 2D Array(2D array=w3756) -> (transposed array=w3763:i16[][])
                    n2203 = Divide(x=w3761, y=w3760) -> (x/y=w3762:dbl)
                    n2204 = Reshape Array(w3763, w3762) -> (w3759:i16[])
                  }
                }
                n2205 = Index Array(array=w3685, index=1) -> (element=w3688:waveform(dbl))
                n2206 = Index Array(array=w3685, index=0) -> (element=w3690:waveform(dbl))
                n2207 = Unbundle By Name(w3688) -> ("Y"=w3692:dbl[])
                n2208 = Unbundle By Name(w3690) -> ("Y"=w3700:dbl[])
                n2209 = case "Write trap pos. data" shown="True" w3666 {
                  tunnel: w3665 -> [_ w3748]
                  tunnel: w3661 -> [_ w3747]
                  frame False {
                  }
                  frame True {
                    n2210 = Write to Binary File(file (use dialog)=w3748, data=w3747, 5:FALSE ("prepend array or string size? (T)"), 9:T30."big-endian, network order" ("byte order (0:big-endian, network order)")) -> ()  [unwired: 1 in, 4 out]
                  }
                }
                n2211 = Write to Binary File(file (use dialog)=w3726, data=w3719, 5:FALSE ("prepend array or string size? (T)"), 9:T30."big-endian, network order" ("byte order (0:big-endian, network order)")) -> ()  [unwired: 1 in, 4 out]
                n2212 = feedback #26(w3692) -> (w3694:dbl[])
                n2213 = Build Array (concatenate)(w3694, w3692) -> (w3693:dbl[])
                n2214 = Select(t=w3692, s=w3668, f=w3693) -> (s? t:f=w3678:dbl[])
                n2215 = feedback-in #26(w3678) -> ()
                n2216 = feedback #27(w3700) -> (w3713:dbl[])
                n2217 = Build Array (concatenate)(w3713, w3700) -> (w3712:dbl[])
                n2218 = Select(t=w3700, s=w3668, f=w3712) -> (s? t:f=w3687:dbl[])
                n2219 = feedback-in #27(w3687) -> ()
                n2220 = Divide(x=w3727, y=w3728) -> (x/y=w3730:dbl)
                n2221 = Multiply(x=w3730, y=100.0) -> (x*y=w3729:dbl)
                n2222 = Build Array(w3687, w3678) -> (→"Saved APD":dbl[][])
                n2223 = Array Size(array=w3687) -> (size(s)=w3705:i32)
                n2224 = Unbundle By Name(w3707) -> ("Y"=w3711:dbl[])
                n2225 = Subtract(x=w3705, y="N pts to average") -> (x-y=w3681:i32)
                n2226 = Multiply(x="N pts to average", y=u16 2) -> (x*y=w3682:u16)
                n2227 = Subtract(x=w3705, y=w3682) -> (x-y=w3680:i32)
                n2228 = feedback #28(w3711) -> (w3710:dbl[])
                n2229 = Build Array (concatenate)(w3710, w3711) -> (w3709:dbl[])
                n2230 = Select(t=w3711, s=w3668, f=w3709) -> (s? t:f=w3708:dbl[])
                "Trap Delta Graph" <- w3708
                n2231 = feedback-in #28(w3708) -> ()
                n2232 = Array Subset(array=w3687, index=w3681, length="N pts to average") -> (w3704:dbl[])
                n2233 = Array Subset(array=w3687, index=w3680, length="N pts to average") -> (w3703:dbl[])
                n2234 = Array Subset(array=w3678, index=w3681, length="N pts to average") -> (w3684:dbl[])
                n2235 = Array Subset(array=w3678, index=w3680, length="N pts to average") -> (w3683:dbl[])
                n2236 = call-poly <vilib>:"Mean.vi"("X"=w3704) -> ("mean"=w3702:dbl)  [unwired: 1 out]
                n2237 = call-poly <vilib>:"Mean.vi"("X"=w3684) -> ("mean"=w3677:dbl)  [unwired: 1 out]
                n2238 = call-poly <vilib>:"Mean.vi"("X"=w3703) -> ("mean"=w3701:dbl)  [unwired: 1 out]
                n2239 = call-poly <vilib>:"Mean.vi"("X"=w3683) -> ("mean"=w3676:dbl)  [unwired: 1 out]
                n2240 = Subtract(x=w3677, y=w3676) -> (x-y=w3667:dbl)
                "Delta Fl. 2" <- w3667
                n2241 = Subtract(x=w3702, y=w3701) -> (x-y=w3699:dbl)
                "Delta Fl. 1" <- w3699
                n2242 = Initialize Array(w3699, 1 ("dimension size")) -> (w3696:dbl[])
                n2243 = Initialize Array(w3667, 1 ("dimension size")) -> (w3673:dbl[])
                n2244 = feedback #29(w3696) -> (w3697:dbl[])
                n2245 = Build Array (concatenate)(w3697, w3696) -> (w3695:dbl[])
                n2246 = feedback #30(w3673) -> (w3674:dbl[])
                n2247 = Build Array (concatenate)(w3674, w3673) -> (w3672:dbl[])
                n2248 = Select(t=w3696, s=w3668, f=w3695) -> (s? t:f=w3671:dbl[])
                n2249 = feedback-in #29(w3671) -> ()
                n2250 = Select(t=w3673, s=w3668, f=w3672) -> (s? t:f=w3670:dbl[])
                n2251 = feedback-in #30(w3670) -> ()
                n2252 = Build Array(w3671, w3670) -> (→"Save APD Deriv":dbl[][])
              }
            }
            "Progress" <- w3644
            "Progress 2" <- w3644
          }
        }
      }
    }
    n2253 = Bundle By Name(cluster=w2338, "Green FB Ch 0"=w2337, "Green FB Ch 1"=w2336) -> (w2320:T49)
    "Green FB Signals (V)" <- w2320
    n2254 = Unbundle By Name(w2320) -> ("Green FB Ch 2"=→"Green FB Plot":dbl)
    n2255 = local read "wait to reset values"() -> (w2406:bool)
    n2256 = Not(x=w2403) -> (.not. x?=w2407:bool)
    n2257 = And(x=w2407, y=w2406) -> (x .and. y?=w2408:bool)
    n2258 = case "Part of MCL raster scanning: returns to initial positions after scan done" shown="False" w2408 {
      tunnel: w2411 -> [w3196 w3203]
      tunnel: [w3196 w3202] -> w2410
      tunnel: w2405 -> [w3195 w3201]
      tunnel: [w3195 w3200] -> w2404
      frame False {
      }
      frame True {
        w3211 = 10.0 ("y")
        w3210 = 32767.0 ("y")
        # "to return scan values\nafter a synchronous \nAOM scan"
        n2259 = local read "AO2"() -> (w3204:dbl)
        n2260 = local read "AO1"() -> (w3205:dbl)
        n2261 = local write "wait to reset values"(FALSE ("wait to reset values")) -> ()
        n2262 = Multiply(x=w3205, y=w3210) -> (x*y=w3207:dbl)
        n2263 = Multiply(x=w3204, y=w3210) -> (x*y=w3209:dbl)
        n2264 = Divide(x=w3207, y=w3211) -> (x/y=w3206:dbl)
        n2265 = Divide(x=w3209, y=w3211) -> (x/y=w3208:dbl)
        n2266 = To Word Integer(number=w3206) -> (16bit integer=w3212:i16)
        n2267 = To Word Integer(number=w3208) -> (16bit integer=w3213:i16)
        n2268 = local read "Total Counts (ticks)"() -> (w3197:u32)
        n2269 = xnode "Read/Write Control"("FPGA VI Reference In"=w3203, "error in"=w3201, "AO1"=w3212, "AO2"=w3213, "MCL count"=w3197) -> ("FPGA VI Reference Out"=w3202:T20, "error out"=w3200:errorcluster)
        n2270 = local read "Scan Range (V)\n(of steps)"() -> (w3198:dbl)
        n2271 = property on="Scan Range (V)\n(of steps)" class="DigNum (strict)"("Val(Sgnl)"=w3198) -> ()  [unwired: 2 in, 2 out]
      }
    }
    n2272 = node-c288() -> ()  [unwired: 2 out]
  }
  n2273 = node-c288(3 ("Processor")) -> (w94:T25)  [unwired: 3 out]
  n2274 = timed-loop "Oscillate AOD (debugging)" {
    tunnel: w44 -> [w3772]
    tunnel: [w3771] -> w56
    timing: w94 -> [_]
    timing-out: [_] -> w93
    stop <- w3771 stop-if-true
    n2275 = node-c288() -> ()  [unwired: 2 out]
    n2276 = event shown="[0] \"Oscillate Set 2\", \"Fish for Tether\": Value Change" {
      selector: _ -> [_ _ _]
      dyn-events: _ -> [_ _ _]
      timeout: _ -> [_ _ _]
      tunnel: w3772 -> [w3779 _ _]
      tunnel: [FALSE ("Stop All") _ w4047] -> w3771
      event "Oscillate Set 2", "Fish for Tether": Value Change {
        n2277 = event-data() -> ()  [unwired: 6 out]
        n2278 = local read "Oscillate Set 2"() -> (w3778:bool)
        n2279 = Or(x=w3778, y="Fish for Tether") -> (x .or. y?=w3776:bool)
        n2280 = case shown="True" w3776 {
          tunnel: w3779 -> [_ w3782]
          tunnel: "Fish for Tether" -> [_ w3781]
          frame False {
          }
          frame True {
            n2281 = case shown="True" w3781 {
              frame False {
              }
              frame True {
                n2282 = local write "Scan axis 2"(TRUE) -> ()
                n2283 = local write "Tether"(FALSE ("Tether")) -> ()
              }
            }
            n2284 = node-c288("Period") -> (w3784:T25)  [unwired: 3 out]
            n2285 = timed-loop "Oscillate AOD" {
              timing: w3784 -> [_]
              timing-out: [_] -> w3783
              tunnel: w3782 -> [w3794]
              tunnel: w3781 -> [w3793]
              i -> [w3796]
              stop <- w3792 stop-if-true
              n2286 = node-c288() -> (w3795:i64)  [unwired: 1 out]
              n2287 = flat-sequence {
                tunnel: w3796 -> [w3822]
                tunnel: w3795 -> [w3821]
                tunnel: w3794 -> [w3805]
                tunnel: w3793 -> [w3807]
                tunnel: [w3807] -> w3791
                tunnel: [w3806] -> w3790
                tunnel: [w3804] -> w3789
                tunnel: [w3801] -> w3787
                tunnel: w3791 -> [w3858]
                tunnel: w3790 -> [w3856]
                tunnel: w3789 -> [w3855]
                tunnel: [w3854] -> w3788
                tunnel: w3787 -> [w3853]
                tunnel: [w3922] -> w3792
                tunnel: w3788 -> [w3920]
                frame #0 {
                  n2288 = Divide(x=w3821, y=i64 1000) -> (x/y=w3816:dbl)
                  n2289 = Multiply(x=w3816, y=w3822) -> (x*y=w3818:dbl)
                  n2290 = Multiply(x="Osc. freq. (Hz)", y=6.283185307179586) -> (x*y=w3819:dbl)
                  n2291 = Multiply(x=w3819, y=w3818) -> (x*y=w3803:dbl)
                  n2292 = local read "BD 1 Frequency 2 (MHz)"() -> (w3800:dbl)
                  n2293 = local read "BD 1 Frequency 1 (MHz)"() -> (w3797:dbl)
                  n2294 = case shown="True" w3807 {
                    tunnel: w3803 -> [w3828 w3835]
                    tunnel: w3800 -> [_ w3845]
                    tunnel: [w3825 w3829] -> w3808
                    tunnel: [FALSE w3838] -> w3804
                    tunnel: [0.0 w3831] -> w3801
                    tunnel: w3797 -> [_ w3830]
                    frame False {
                      n2295 = Sine(x=w3828) -> (sin(x)=w3826:dbl)
                      n2296 = Multiply(x=w3826, y="Osc. amp. (MHz)") -> (x*y=w3825:dbl)
                    }
                    frame True {
                      n2297 = Cosine(x=w3835) -> (cos(x)=w3848:dbl)
                      n2298 = Subtract(x=w3845, y=w3830) -> (x-y=w3844:dbl)
                      n2299 = Decrement(x=w3848) -> (x-1=w3847:dbl)
                      n2300 = Subtract(x=w3844, y="Closest Delta (MHz)") -> (x-y=w3841:dbl)
                      n2301 = Divide(x=w3847, y=2.0) -> (x/y=w3842:dbl)
                      n2302 = Multiply(x=w3842, y=w3841) -> (x*y=w3829:dbl)
                      n2303 = local read "Vec Mean of T1 T2"() -> (w3837:dbl[])
                      n2304 = Greater?(x=w3837, y="Stop F (pN)") -> (0:w3839:bool[])
                      n2305 = Or Array Elements(Boolean array=w3839) -> (logical OR=w3838:bool)
                      n2306 = Divide(x=w3835, y=6.283185307179586) -> (x/y=w3834:dbl)
                      n2307 = Round Toward +Infinity(x=w3834) -> (ceil(x): smallest int >= x=w3831:dbl)
                      "Attempts" <- w3831
                      n2308 = Greater?(x=w3831, y="Attempt Limit") -> (0:w3833:bool)
                      n2309 = case shown="True" w3833 {
                        frame False {
                        }
                        frame True {
